vi "Initalize_33522b&2400&Delta_lxy.vi"(4 "Delta Mode Params In":T9={"High Level (A)"=0.001, "Low Level (A)"=-0.001, "Delay (s)"=0.002, "Num Cycles Mode"=enum."Finite Count", "Finite Count"=10, "Abort On\nCompliance?"=FALSE, "Cold Swithing\nMode Enabled?"=FALSE} {"Finite Count" min=1 max=65536; "Low Level (A)" min=-0.105 max=0.0 format="%.3p"; "High Level (A)" min=0.0 max=0.105 format="%.3p"; "Delay (s)" min=0.001 max=9999.999 format="%.3f"}, 5 "Output Level (0)":dbl=0.001, 6 "2812 -A Params In":T20={"Auto Range?"=FALSE, "Man / Selected\nRange"=enum."10mV", "Enable Digital\nFilter?"=FALSE, "Filter Type"=enum."Moving", "Filter Count"=10, "Filter\nWindow (%)"=0.01, "Enable Analog\nFilter?"=FALSE, "NPLCs"=5} {"Filter\nWindow (%)" min=0.0 max=10.0 step=0.01 format="%.2f"; "Filter Count" min=1 max=100; "NPLCs" min=1 max=10}, 7 "Compliance  Level (0.1)":dbl=10.0, 8 "error in (no error)":errorcluster, 11 "config":T1={"initialize"=enum."SR830", "6221"={"6221 Resource"="GPIB0::24::INSTR", "Delta status"=FALSE, "电流|RMS(A)"=0.0}, "SR830+6221"={"source"=0, "Current(A)"=0.0, "阻抗(Ohm)"=0.0, "SR830 1"=FALSE, "SR830 2"=FALSE, "SR830 3"=FALSE, "SR830 4"=FALSE, "VISA 1"="", "VISA 2"="", "VISA 3"="", "VISA 4"="", "Reserve 1"=0, "Reserve 2"=-1, "Reserve 3"=-1, "Reserve 4"=-1, "Sensitivity 1"=-1, "Sensitivity 2"=0, "Sensitivity 3"=-1, "Sensitivity 4"=-1, "量程入 1"=0, "量程入 2"=0, "量程入 3"=0, "量程入 4"=0}, "2400"={"2400"=FALSE, "VISA"="GPIB0::9::INSTR", "Output Level (0)"=1e-05, "Compliance  Level (0.1)"=10.0, "ch"=[]}, "ch"={"ch"=[], "current"=[], "change?"=[], "holding current\nwhen change ch?"=FALSE, "current offset"=[]}, "Instrument"={"limit"={"Field limit"=0.0, "Field rate limit"=0.0, "Temp limit"=0.0, "Temp low limit"=0.0, "Temp rate limit "=0.0}, "genarl"={"行数"=refnum, "编辑列表框？"=refnum, "列表框"=refnum, "camg 振荡状态"=refnum, "Aborting"=refnum, "数据文件"=refnum, "warning"=refnum, "vi路径"="", "Instrument Type"=enum."PPMS-Rotate"}, "cmag"={"TM620"="TCPIP0::192.168.1.5::4266::SOCKET", "M24C Resource"="GPIB0::24::INSTR", "4G supply"="", "Temp Status 24C"=refnum, "Temp"=refnum, "9T信号"=refnum, "4g supply status"=refnum, "in-plane"="", "out-plane"="", "in-plane signal"=FALSE, "out-plane signal"=FALSE, "in plane 信号"=refnum, "pzt volt"=refnum, "camg Rate"=refnum}, "lengtou2"={"750 visa"="", "750 rotate"="", "semaphore 340"=refnum, "semaphore 750"=refnum, "750 field status"=refnum, "Input (0:A) 340"=0, "340 Resource"="GPIB0::14::INSTR", "340 Status"=refnum, "Input (0:B) 340"=1, "Loop (0: 1)"=0, "Loop (1: 1)"=0, "TCP master instance"=refnum}, "lengtou"={"TCP master instance"=refnum, "335 Status"=refnum, "335 Resource "="GPIB0::24::INSTR", "Input (0:A) 335"=0, "Input (0:B) 335"=1, "Heater Output (1:1) 335"=1, "semaphore 335"=refnum}, "325 for test"={"quantum design"=refnum, "semaphore 325"=refnum, "325 Resource "="GPIB0::13::INSTR", "Input (0:A) 325"=0, "Heater Output (1:1) 325"=1, "325 Status"=refnum}}, "2614B"={"2614B chA"=FALSE, "2614B chB"=FALSE, "VISA"=""}, "33522b"={"33522b resource name"="GPIB0::16::INSTR", "零电压"=0.0, "最大电压"=148.0, "间隔"=4.0, "最小电压"=-48.0, "loop"=0.0}, "gating type"=enum."2614(daul)", "层数"=0, "行数"=0, "是否处理"=[], "current 2"=[]} {"Instrument"."325 for test"."Heater Output (1:1) 325" items=["1"=1, "2"=2]; "Instrument"."325 for test"."Input (0:A) 325" items=["A", "B"]; "Instrument"."lengtou"."Heater Output (1:1) 335" items=["1"=1, "2"=2]; "Instrument"."lengtou"."Input (0:B) 335" items=["A", "B"]; "Instrument"."lengtou"."Input (0:A) 335" items=["A", "B"]; "Instrument"."lengtou2"."Loop (1: 1)" items=["1", "2"]; "Instrument"."lengtou2"."Loop (0: 1)" items=["1", "2"]; "Instrument"."lengtou2"."Input (0:B) 340" items=["A", "B", "C", "D"]; "Instrument"."lengtou2"."Input (0:A) 340" items=["A", "B", "C", "D"]; "SR830+6221"."Sensitivity 4" items=["Auto Gain"=-1, "2 nV/fA"=0, "5 nV/fA"=1, "10 nV/fA"=2, "20 nV/fA"=3, "50 nV/fA"=4, "100 nV/fA"=5, "200 nV/fA"=6, "500 nV/fA"=7, "1 uV/pA"=8, "2 uV/pA"=9, "5 uV/pA"=10, "10 uV/pA"=11, "20 uV/pA"=12, "50 uV/pA"=13, "100 uV/pA"=14, "200 uV/pA"=15, "500 uV/pA"=16, "1 mV/nA"=17, "2 mV/nA"=18, "5 mV/nA"=19, "10 mV/nA"=20, "20 mV/nA"=21, "50 mV/nA"=22, "100 mV/nA"=23, "200 mV/nA"=24, "500 mV/mA"=25, "1 V/uA"=26]; "SR830+6221"."Sensitivity 3" items=["Auto Gain"=-1, "2 nV/fA"=0, "5 nV/fA"=1, "10 nV/fA"=2, "20 nV/fA"=3, "50 nV/fA"=4, "100 nV/fA"=5, "200 nV/fA"=6, "500 nV/fA"=7, "1 uV/pA"=8, "2 uV/pA"=9, "5 uV/pA"=10, "10 uV/pA"=11, "20 uV/pA"=12, "50 uV/pA"=13, "100 uV/pA"=14, "200 uV/pA"=15, "500 uV/pA"=16, "1 mV/nA"=17, "2 mV/nA"=18, "5 mV/nA"=19, "10 mV/nA"=20, "20 mV/nA"=21, "50 mV/nA"=22, "100 mV/nA"=23, "200 mV/nA"=24, "500 mV/mA"=25, "1 V/uA"=26]; "SR830+6221"."Sensitivity 1" items=["Auto Gain"=-1, "2 nV/fA"=0, "5 nV/fA"=1, "10 nV/fA"=2, "20 nV/fA"=3, "50 nV/fA"=4, "100 nV/fA"=5, "200 nV/fA"=6, "500 nV/fA"=7, "1 uV/pA"=8, "2 uV/pA"=9, "5 uV/pA"=10, "10 uV/pA"=11, "20 uV/pA"=12, "50 uV/pA"=13, "100 uV/pA"=14, "200 uV/pA"=15, "500 uV/pA"=16, "1 mV/nA"=17, "2 mV/nA"=18, "5 mV/nA"=19, "10 mV/nA"=20, "20 mV/nA"=21, "50 mV/nA"=22, "100 mV/nA"=23, "200 mV/nA"=24, "500 mV/mA"=25, "1 V/uA"=26]; "SR830+6221"."Sensitivity 2" items=["Auto Gain"=-1, "2 nV/fA"=0, "5 nV/fA"=1, "10 nV/fA"=2, "20 nV/fA"=3, "50 nV/fA"=4, "100 nV/fA"=5, "200 nV/fA"=6, "500 nV/fA"=7, "1 uV/pA"=8, "2 uV/pA"=9, "5 uV/pA"=10, "10 uV/pA"=11, "20 uV/pA"=12, "50 uV/pA"=13, "100 uV/pA"=14, "200 uV/pA"=15, "500 uV/pA"=16, "1 mV/nA"=17, "2 mV/nA"=18, "5 mV/nA"=19, "10 mV/nA"=20, "20 mV/nA"=21, "50 mV/nA"=22, "100 mV/nA"=23, "200 mV/nA"=24, "500 mV/mA"=25, "1 V/uA"=26]; "SR830+6221"."Reserve 4" items=["Auto Gain"=-1, "2 nV/fA"=0, "5 nV/fA"=1, "10 nV/fA"=2, "20 nV/fA"=3, "50 nV/fA"=4, "100 nV/fA"=5, "200 nV/fA"=6, "500 nV/fA"=7, "1 uV/pA"=8, "2 uV/pA"=9, "5 uV/pA"=10, "10 uV/pA"=11, "20 uV/pA"=12, "50 uV/pA"=13, "100 uV/pA"=14, "200 uV/pA"=15, "500 uV/pA"=16, "1 mV/nA"=17, "2 mV/nA"=18, "5 mV/nA"=19, "10 mV/nA"=20, "20 mV/nA"=21, "50 mV/nA"=22, "100 mV/nA"=23, "200 mV/nA"=24, "500 mV/mA"=25, "1 V/uA"=26]; "SR830+6221"."Reserve 3" items=["Auto Reserve"=-1, "High Reserve"=0, "Normal"=1, "Low Noise"=2]; "SR830+6221"."Reserve 2" items=["Auto Reserve"=-1, "High Reserve"=0, "Normal"=1, "Low Noise"=2]; "SR830+6221"."Reserve 1" items=["Auto Reserve"=-1, "High Reserve"=0, "Normal"=1, "Low Noise"=2]; "SR830+6221"."source" items=["SR830 1", "SR830 2", "SR830 3", "SR830 4"]}) -> (0 "输出簇":T1={"initialize"=enum."SR830", "6221"={"6221 Resource"="GPIB0::24::INSTR", "Delta status"=FALSE, "电流|RMS(A)"=0.0}, "SR830+6221"={"source"=0, "Current(A)"=0.0, "阻抗(Ohm)"=0.0, "SR830 1"=FALSE, "SR830 2"=FALSE, "SR830 3"=FALSE, "SR830 4"=FALSE, "VISA 1"="", "VISA 2"="", "VISA 3"="", "VISA 4"="", "Reserve 1"=0, "Reserve 2"=-1, "Reserve 3"=-1, "Reserve 4"=-1, "Sensitivity 1"=-1, "Sensitivity 2"=0, "Sensitivity 3"=-1, "Sensitivity 4"=-1, "量程入 1"=0, "量程入 2"=0, "量程入 3"=0, "量程入 4"=0}, "2400"={"2400"=FALSE, "VISA"="", "Output Level (0)"=1e-05, "Compliance  Level (0.1)"=10.0, "ch"=[]}, "ch"={"ch"=[], "current"=[], "change?"=[], "holding current\nwhen change ch?"=FALSE, "current offset"=[]}, "Instrument"={"limit"={"Field limit"=0.0, "Field rate limit"=0.0, "Temp limit"=0.0, "Temp low limit"=0.0, "Temp rate limit "=0.0}, "genarl"={"行数"=refnum, "编辑列表框？"=refnum, "列表框"=refnum, "camg 振荡状态"=refnum, "Aborting"=refnum, "数据文件"=refnum, "warning"=refnum, "vi路径"="", "Instrument Type"=enum."PPMS-Rotate"}, "cmag"={"TM620"="TCPIP0::192.168.1.5::4266::SOCKET", "M24C Resource"="GPIB0::24::INSTR", "4G supply"="", "Temp Status 24C"=refnum, "Temp"=refnum, "9T信号"=refnum, "4g supply status"=refnum, "in-plane"="", "out-plane"="", "in-plane signal"=FALSE, "out-plane signal"=FALSE, "in plane 信号"=refnum, "pzt volt"=refnum, "camg Rate"=refnum}, "lengtou2"={"750 visa"="", "750 rotate"="", "semaphore 340"=refnum, "semaphore 750"=refnum, "750 field status"=refnum, "Input (0:A) 340"=0, "340 Resource"="GPIB0::14::INSTR", "340 Status"=refnum, "Input (0:B) 340"=1, "Loop (0: 1)"=0, "Loop (1: 1)"=0, "TCP master instance"=refnum}, "lengtou"={"TCP master instance"=refnum, "335 Status"=refnum, "335 Resource "="GPIB0::24::INSTR", "Input (0:A) 335"=0, "Input (0:B) 335"=1, "Heater Output (1:1) 335"=1, "semaphore 335"=refnum}, "325 for test"={"quantum design"=refnum, "semaphore 325"=refnum, "325 Resource "="GPIB0::13::INSTR", "Input (0:A) 325"=0, "Heater Output (1:1) 325"=1, "325 Status"=refnum}}, "2614B"={"2614B chA"=FALSE, "2614B chB"=FALSE, "VISA"=""}, "33522b"={"33522b resource name"="", "零电压"=0.0, "最大电压"=148.0, "间隔"=4.0, "最小电压"=-48.0, "loop"=0.0}, "gating type"=enum."2614(daul)", "层数"=0, "行数"=0, "是否处理"=[], "current 2"=[]} {"Instrument"."325 for test"."Heater Output (1:1) 325" items=["1"=1, "2"=2]; "Instrument"."325 for test"."Input (0:A) 325" items=["A", "B"]; "Instrument"."lengtou"."Heater Output (1:1) 335" items=["1"=1, "2"=2]; "Instrument"."lengtou"."Input (0:B) 335" items=["A", "B"]; "Instrument"."lengtou"."Input (0:A) 335" items=["A", "B"]; "Instrument"."lengtou2"."Loop (1: 1)" items=["1", "2"]; "Instrument"."lengtou2"."Loop (0: 1)" items=["1", "2"]; "Instrument"."lengtou2"."Input (0:B) 340" items=["A", "B", "C", "D"]; "Instrument"."lengtou2"."Input (0:A) 340" items=["A", "B", "C", "D"]; "SR830+6221"."Sensitivity 4" items=["Auto Gain"=-1, "2 nV/fA"=0, "5 nV/fA"=1, "10 nV/fA"=2, "20 nV/fA"=3, "50 nV/fA"=4, "100 nV/fA"=5, "200 nV/fA"=6, "500 nV/fA"=7, "1 uV/pA"=8, "2 uV/pA"=9, "5 uV/pA"=10, "10 uV/pA"=11, "20 uV/pA"=12, "50 uV/pA"=13, "100 uV/pA"=14, "200 uV/pA"=15, "500 uV/pA"=16, "1 mV/nA"=17, "2 mV/nA"=18, "5 mV/nA"=19, "10 mV/nA"=20, "20 mV/nA"=21, "50 mV/nA"=22, "100 mV/nA"=23, "200 mV/nA"=24, "500 mV/mA"=25, "1 V/uA"=26]; "SR830+6221"."Sensitivity 3" items=["Auto Gain"=-1, "2 nV/fA"=0, "5 nV/fA"=1, "10 nV/fA"=2, "20 nV/fA"=3, "50 nV/fA"=4, "100 nV/fA"=5, "200 nV/fA"=6, "500 nV/fA"=7, "1 uV/pA"=8, "2 uV/pA"=9, "5 uV/pA"=10, "10 uV/pA"=11, "20 uV/pA"=12, "50 uV/pA"=13, "100 uV/pA"=14, "200 uV/pA"=15, "500 uV/pA"=16, "1 mV/nA"=17, "2 mV/nA"=18, "5 mV/nA"=19, "10 mV/nA"=20, "20 mV/nA"=21, "50 mV/nA"=22, "100 mV/nA"=23, "200 mV/nA"=24, "500 mV/mA"=25, "1 V/uA"=26]; "SR830+6221"."Sensitivity 1" items=["Auto Gain"=-1, "2 nV/fA"=0, "5 nV/fA"=1, "10 nV/fA"=2, "20 nV/fA"=3, "50 nV/fA"=4, "100 nV/fA"=5, "200 nV/fA"=6, "500 nV/fA"=7, "1 uV/pA"=8, "2 uV/pA"=9, "5 uV/pA"=10, "10 uV/pA"=11, "20 uV/pA"=12, "50 uV/pA"=13, "100 uV/pA"=14, "200 uV/pA"=15, "500 uV/pA"=16, "1 mV/nA"=17, "2 mV/nA"=18, "5 mV/nA"=19, "10 mV/nA"=20, "20 mV/nA"=21, "50 mV/nA"=22, "100 mV/nA"=23, "200 mV/nA"=24, "500 mV/mA"=25, "1 V/uA"=26]; "SR830+6221"."Sensitivity 2" items=["Auto Gain"=-1, "2 nV/fA"=0, "5 nV/fA"=1, "10 nV/fA"=2, "20 nV/fA"=3, "50 nV/fA"=4, "100 nV/fA"=5, "200 nV/fA"=6, "500 nV/fA"=7, "1 uV/pA"=8, "2 uV/pA"=9, "5 uV/pA"=10, "10 uV/pA"=11, "20 uV/pA"=12, "50 uV/pA"=13, "100 uV/pA"=14, "200 uV/pA"=15, "500 uV/pA"=16, "1 mV/nA"=17, "2 mV/nA"=18, "5 mV/nA"=19, "10 mV/nA"=20, "20 mV/nA"=21, "50 mV/nA"=22, "100 mV/nA"=23, "200 mV/nA"=24, "500 mV/mA"=25, "1 V/uA"=26]; "SR830+6221"."Reserve 4" items=["Auto Gain"=-1, "2 nV/fA"=0, "5 nV/fA"=1, "10 nV/fA"=2, "20 nV/fA"=3, "50 nV/fA"=4, "100 nV/fA"=5, "200 nV/fA"=6, "500 nV/fA"=7, "1 uV/pA"=8, "2 uV/pA"=9, "5 uV/pA"=10, "10 uV/pA"=11, "20 uV/pA"=12, "50 uV/pA"=13, "100 uV/pA"=14, "200 uV/pA"=15, "500 uV/pA"=16, "1 mV/nA"=17, "2 mV/nA"=18, "5 mV/nA"=19, "10 mV/nA"=20, "20 mV/nA"=21, "50 mV/nA"=22, "100 mV/nA"=23, "200 mV/nA"=24, "500 mV/mA"=25, "1 V/uA"=26]; "SR830+6221"."Reserve 3" items=["Auto Reserve"=-1, "High Reserve"=0, "Normal"=1, "Low Noise"=2]; "SR830+6221"."Reserve 2" items=["Auto Reserve"=-1, "High Reserve"=0, "Normal"=1, "Low Noise"=2]; "SR830+6221"."Reserve 1" items=["Auto Reserve"=-1, "High Reserve"=0, "Normal"=1, "Low Noise"=2]; "SR830+6221"."source" items=["SR830 1", "SR830 2", "SR830 3", "SR830 4"]}, 3 "33522b resource name":refnum<visa-resource-name>)   [LabVIEW 2019, in "nematic.lvlib"]
uses:
  nematic.lvlib
  lib/Keithley 622x/Configure/2182 -A/Low Level/Typedefs/KE2182 -- Voltage Ranges.ctl
  lib/Keithley 622x/Configure/2182 -A/Low Level/Typedefs/KE2182 -- Filter Type.ctl
  lib/Keithley 622x/Configure/2182 -A/Low Level/Typedefs/KE2182 -- Filter Count.ctl
  lib/Keithley 622x/Configure/2182 -A/Low Level/Typedefs/KE2182 -- Filter Window.ctl
  lib/Keithley 622x/Configure/2182 -A/Low Level/Typedefs/KE2182 -- NPLCs.ctl
  lib/Keithley 622x/Configure/Delta PDelta DCon Modes/Typedefs/KE622x -- Delta Mode Params.ctl
  lib/Keithley 622x/Configure/Delta PDelta DCon Modes/Low Level/Typedefs/KE622x -- Delta PDelta Mode High Level.ctl
  lib/Keithley 622x/Configure/Delta PDelta DCon Modes/Low Level/Typedefs/KE622x -- Delta PDelta Mode Low Level.ctl
  lib/Keithley 622x/Configure/Delta PDelta DCon Modes/Low Level/Typedefs/KE622x -- Delta DCon Mode Delay.ctl
  lib/Keithley 622x/Configure/Delta PDelta DCon Modes/Low Level/Typedefs/KE622x -- Delta PDelta Mode Num Cycles Mode.ctl
  lib/Keithley 622x/Configure/Delta PDelta DCon Modes/Low Level/Typedefs/KE622x -- Delta PDelta Mode Num Cycles.ctl
  ctl/config.ctl
  <vilib>/NI/Modbus Library/API/Master/Modbus Master.lvclass
  ctl/initialize.ctl
  ctl/Instrument.ctl
  ctl/limit.ctl
  ctl/warning.ctl
  ctl/Instrument Type.ctl
  ctl/335 state.ctl
  ctl/9T mag field stauts.ctl
  C:/Users/fuyang/Desktop/postdoctor/labview/labview-measure/lib/QDInstrument.dll
  lib/QDInstrument.dll
  ctl/Gating type.ctl
  lib/Keithley 622x/Configure/Units/Typedefs/KE622x -- Voltage Meas Units.ctl
  lib/Keithley 24XX/Keithley 24XX.lvlib
  lib/Keithley 622x/Keithley 622x.lvlib
panel:
  in  "Init Delta Meas? (T)":bool=TRUE
  in  "Enable Remote Sensing (T: Enable)":bool=TRUE
  in  "Serial Configuration":T8={"Baud Rate"=9600, "Parity"=0, "Data Bits"=8, "Stop Bits"=10, "Flow Control"=0} {"Flow Control" items=["None", "XON/XOFF", "RTS/CTS", "XON/XOFF & RTS/CTS", "DTR/DSR", "XON/XOFF & DTR/DSR"]; "Stop Bits" items=["1.0"=10, "1.5"=15, "2.0"=20]; "Data Bits" items=["7"=7, "8"=8]; "Parity" items=["None", "Odd", "Even", "Mark", "Space"]; "Baud Rate" items=["300"=300, "600"=600, "1200"=1200, "2400"=2400, "4800"=4800, "9600"=9600, "19200"=19200]}
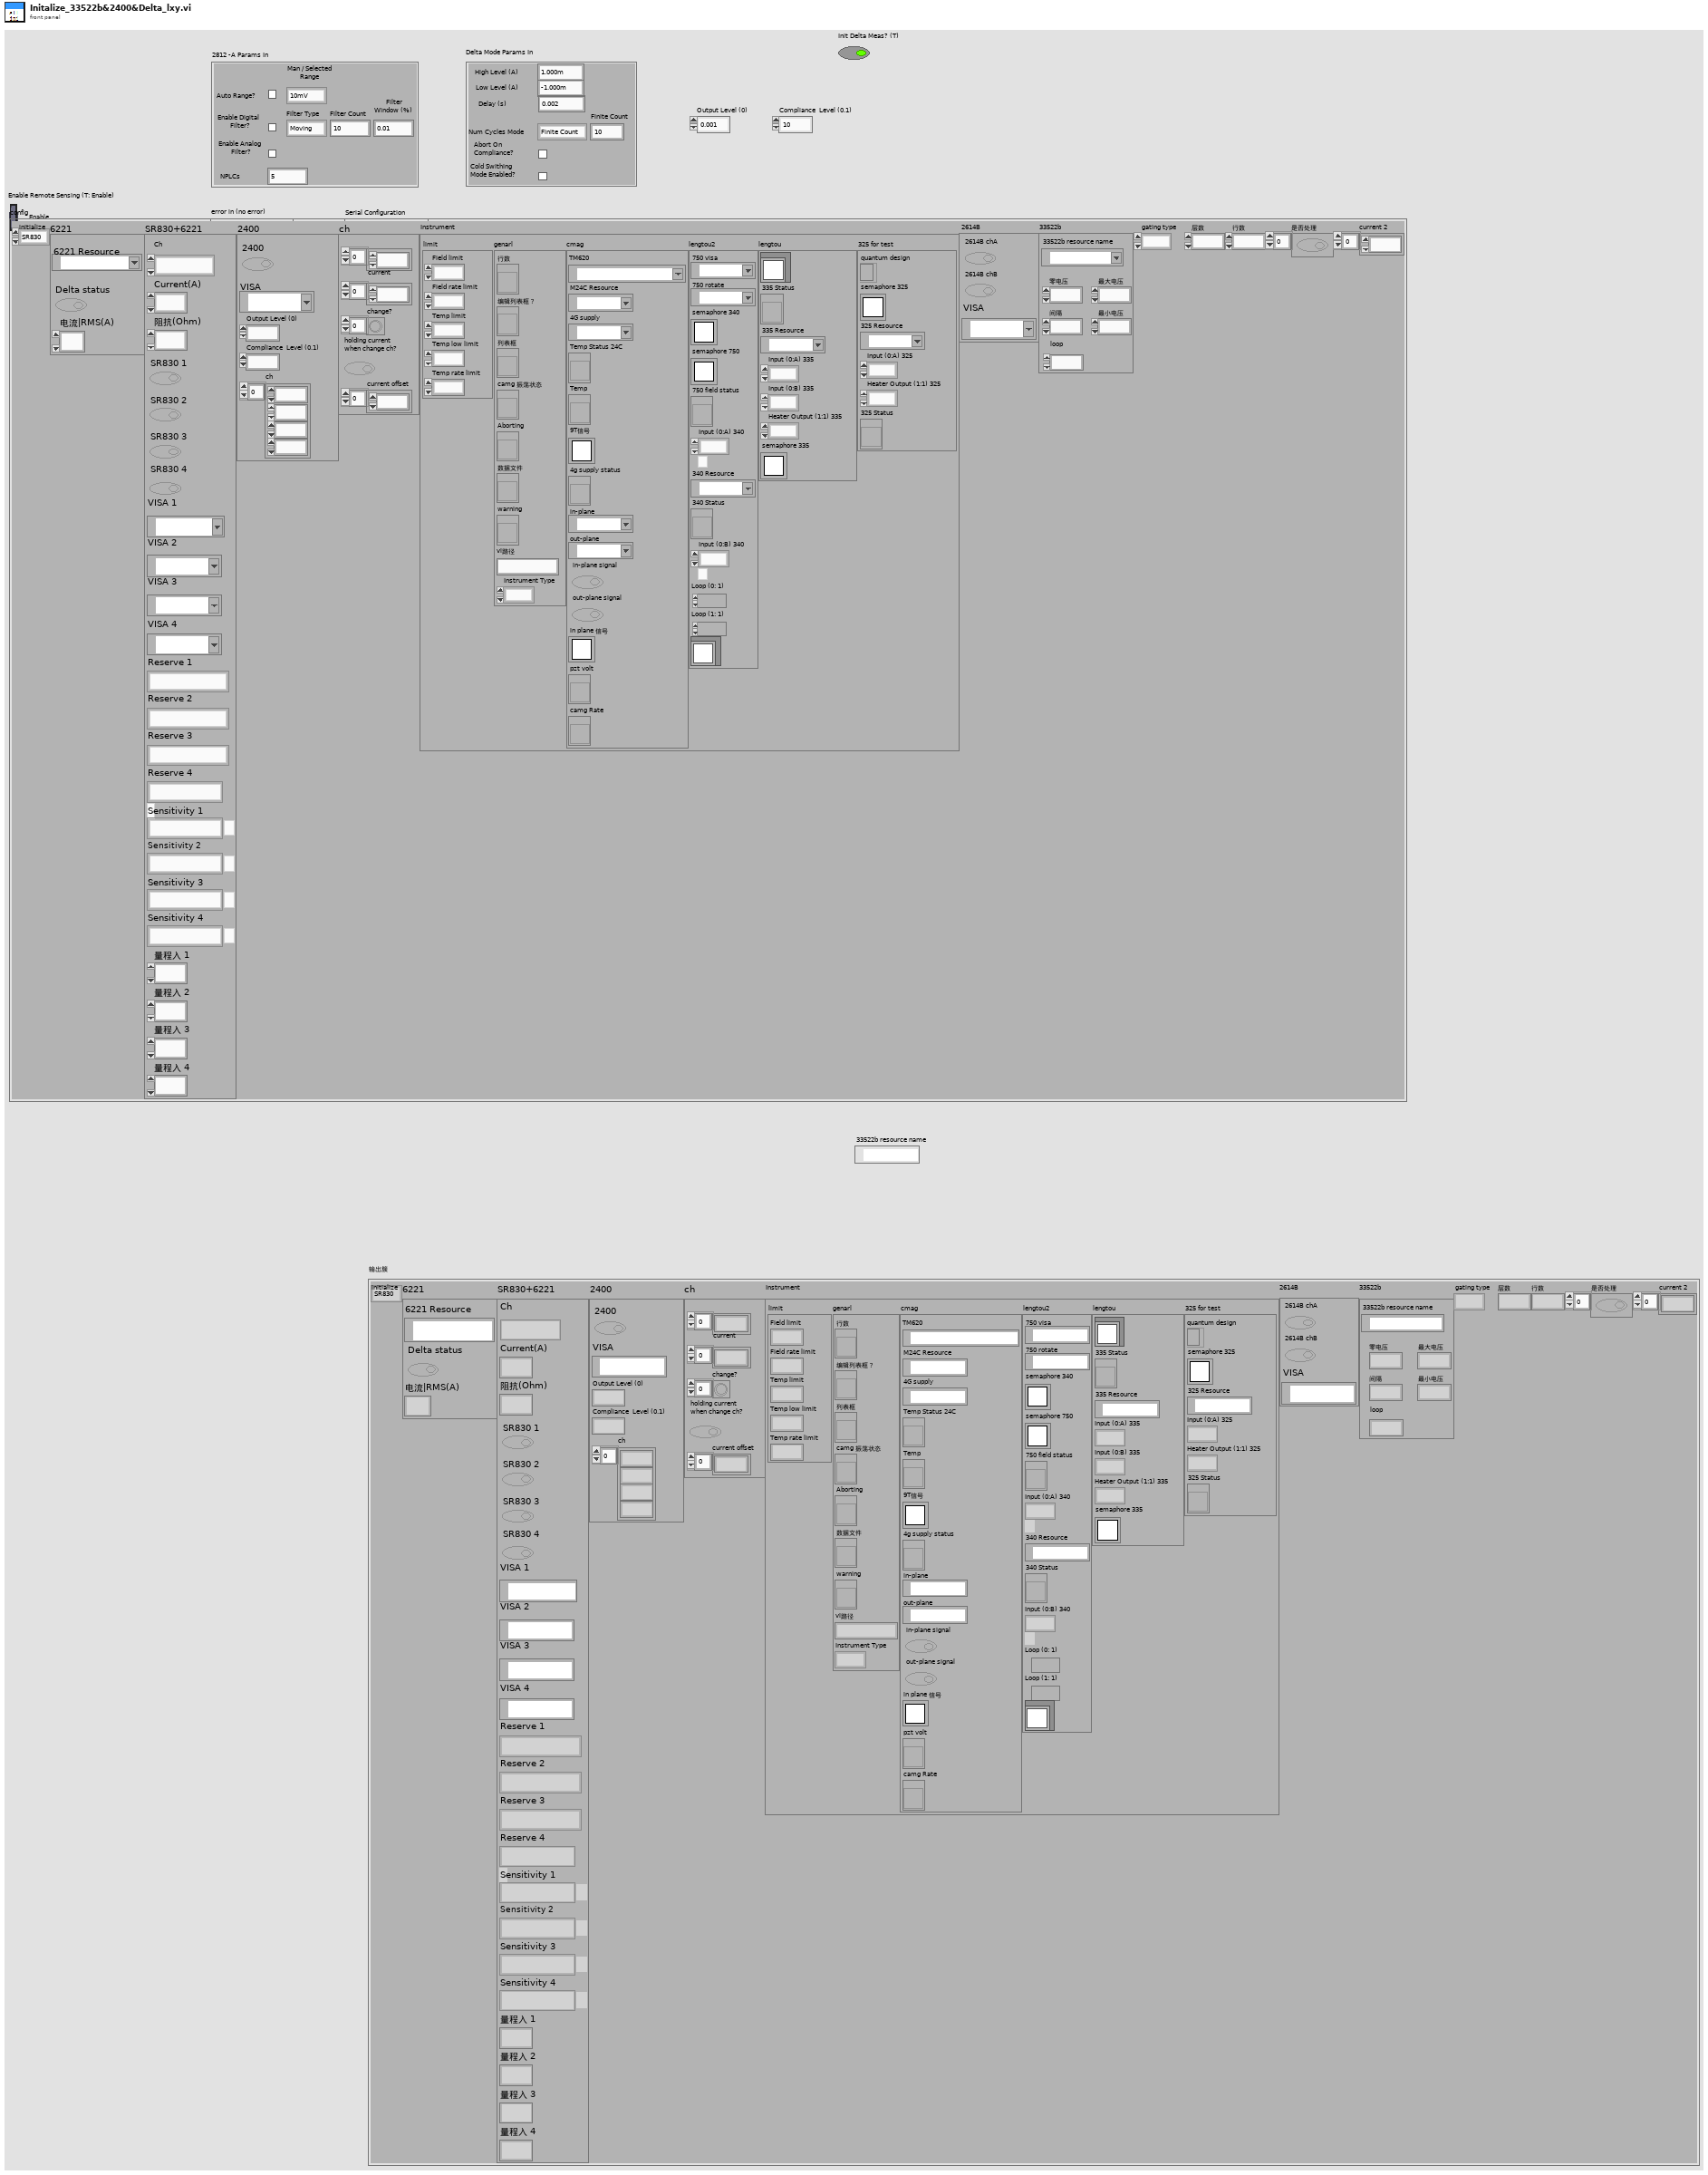
[diagram p1: front panel]
types:
  T1 = typedef "config.ctl" = cluster{"initialize":T2, "6221":cluster{"6221 Resource":refnum<visa-resource-name>, "Delta status":bool, "电流|RMS(A)":dbl}, "SR830+6221":cluster{"source":u16, "Current(A)":dbl, "阻抗(Ohm)":dbl, "SR830 1":bool, "SR830 2":bool, "SR830 3":bool, "SR830 4":bool, "VISA 1":refnum<visa-resource-name>, "VISA 2":refnum<visa-resource-name>, "VISA 3":refnum<visa-resource-name>, "VISA 4":refnum<visa-resource-name>, "Reserve 1":i16, "Reserve 2":i16, "Reserve 3":i16, "Reserve 4":i16, "Sensitivity 1":i16, "Sensitivity 2":i16, "Sensitivity 3":i16, "Sensitivity 4":i16, "量程入 1":i32, "量程入 2":i32, "量程入 3":i32, "量程入 4":i32}, "2400":cluster{"2400":bool, "VISA":refnum<visa-resource-name>, "Output Level (0)":dbl, "Compliance  Level (0.1)":dbl, "ch":i32[]}, "ch":cluster{"ch":i32[], "current":dbl[], "change?":bool[], "holding current\nwhen change ch?":bool, "current offset":dbl[]}, "Instrument":T3, "2614B":cluster{"2614B chA":bool, "2614B chB":bool, "VISA":refnum<visa-resource-name>}, "33522b":cluster{"33522b resource name":refnum<visa-resource-name>, "零电压":dbl, "最大电压":dbl, "间隔":dbl, "最小电压":dbl, "loop":dbl}, "gating type":T7, "层数":i32, "行数":i32, "是否处理":bool[], "current 2":dbl[]}
  T2 = typedef "initialize.ctl" = enum16{"SR830", "keithley6221-SR830", "Delta", "Delta-tunnelling", "keithley6221-2182-DC", "PZT", "4200"}
  T3 = typedef "Instrument.ctl" = cluster{"limit":T4, "genarl":cluster{"行数":refnum<vi>, "编辑列表框？":refnum<vi>, "列表框":refnum<vi>, "camg 振荡状态":refnum<vi>, "Aborting":refnum<vi>, "数据文件":refnum<vi>, "warning":refnum<vi>, "vi路径":string, "Instrument Type":T5}, "cmag":cluster{"TM620":refnum<visa-resource-name>, "M24C Resource":refnum<visa-resource-name>, "4G supply":refnum<visa-resource-name>, "Temp Status 24C":refnum<vi>, "Temp":refnum<vi>, "9T信号":T6, "4g supply status":refnum<vi>, "in-plane":refnum<visa-resource-name>, "out-plane":refnum<visa-resource-name>, "in-plane signal":bool, "out-plane signal":bool, "in plane 信号":T6, "pzt volt":refnum<vi>, "camg Rate":refnum<vi>}, "lengtou2":cluster{"750 visa":refnum<visa-resource-name>, "750 rotate":refnum<visa-resource-name>, "semaphore 340":T6, "semaphore 750":T6, "750 field status":refnum<vi>, "Input (0:A) 340":u16, "340 Resource":refnum<visa-resource-name>, "340 Status":refnum<vi>, "Input (0:B) 340":u16, "Loop (0: 1)":u16, "Loop (1: 1)":u16, "TCP master instance":refnum<class "Modbus Master.lvclass">}, "lengtou":cluster{"TCP master instance":refnum<class "Modbus Master.lvclass">, "335 Status":refnum<vi>, "335 Resource ":refnum<visa-resource-name>, "Input (0:A) 335":u16, "Input (0:B) 335":u16, "Heater Output (1:1) 335":u16, "semaphore 335":T6}, "325 for test":cluster{"quantum design":refnum<k24>, "semaphore 325":T6, "325 Resource ":refnum<visa-resource-name>, "Input (0:A) 325":u16, "Heater Output (1:1) 325":u16, "325 Status":refnum<vi>}}
  T4 = typedef "limit.ctl" = cluster{"Field limit":dbl, "Field rate limit":dbl, "Temp limit":dbl, "Temp low limit":dbl, "Temp rate limit ":dbl}
  T5 = typedef "Instrument Type.ctl" = enum16{"PPMS", "VersaLab", "DynaCool", "SVSM", "PPMS-Rotate", "Lakeshore335", "lengtou2", "9T mag old", "9T cmag", "9T cmag DAC", "9T cmag rotate", "test"}
  T6 = typedef "Semaphore RefNum" = refnum<k1>
  T7 = typedef "Gating type.ctl" = enum32{"null", "2614(daul)", "2400", "6517B"}
  T8 = cluster{"Baud Rate":u32, "Parity":u16, "Data Bits":u16, "Stop Bits":u16, "Flow Control":u16}
  T9 = typedef "Keithley 622x.lvlib/KE622x -- Delta Mode Params.ctl" = cluster{"High Level (A)":T10, "Low Level (A)":T11, "Delay (s)":T12, "Num Cycles Mode":T13, "Finite Count":T14, "Abort On\nCompliance?":bool, "Cold Swithing\nMode Enabled?":bool}
  T10 = typedef "Keithley 622x.lvlib/KE622x -- Delta PDelta Mode High Level.ctl" = dbl
  T11 = typedef "Keithley 622x.lvlib/KE622x -- Delta PDelta Mode Low Level.ctl" = dbl
  T12 = typedef "Keithley 622x.lvlib/KE622x -- Delta DCon Mode Delay.ctl" = dbl
  T13 = typedef "Keithley 622x.lvlib/KE622x -- Delta PDelta Mode Num Cycles Mode.ctl" = enum16{"Finite Count", "Infinite"}
  T14 = typedef "Keithley 622x.lvlib/KE622x -- Delta PDelta Mode Num Cycles.ctl" = u32
  T15 = typedef "Keithley 622x.lvlib/KE2182 -- Voltage Ranges.ctl" = enum16{"10mV", "100mV", "1V", "10V", "100V"}
  T16 = typedef "Keithley 622x.lvlib/KE2182 -- Filter Type.ctl" = enum16{"Moving", "Repeat"}
  T17 = typedef "Keithley 622x.lvlib/KE2182 -- Filter Count.ctl" = u32
  T18 = typedef "Keithley 622x.lvlib/KE2182 -- Filter Window.ctl" = dbl
  T19 = typedef "Keithley 622x.lvlib/KE2182 -- NPLCs.ctl" = u32
  T20 = cluster{"Auto Range?":bool, "Man / Selected\nRange":T15, "Enable Digital\nFilter?":bool, "Filter Type":T16, "Filter Count":T17, "Filter\nWindow (%)":T18, "Enable Analog\nFilter?":bool, "NPLCs":T19}
  T21 = typedef "Keithley 622x.lvlib/KE622x -- Voltage Meas Units.ctl" = enum16{"Volts", "Ohms", "Watts", "Siemens"}
  T22 = typedef "Keithley 622x.lvlib/KE622x -- On Off Control.ctl" = enum16{"Off", "On"}
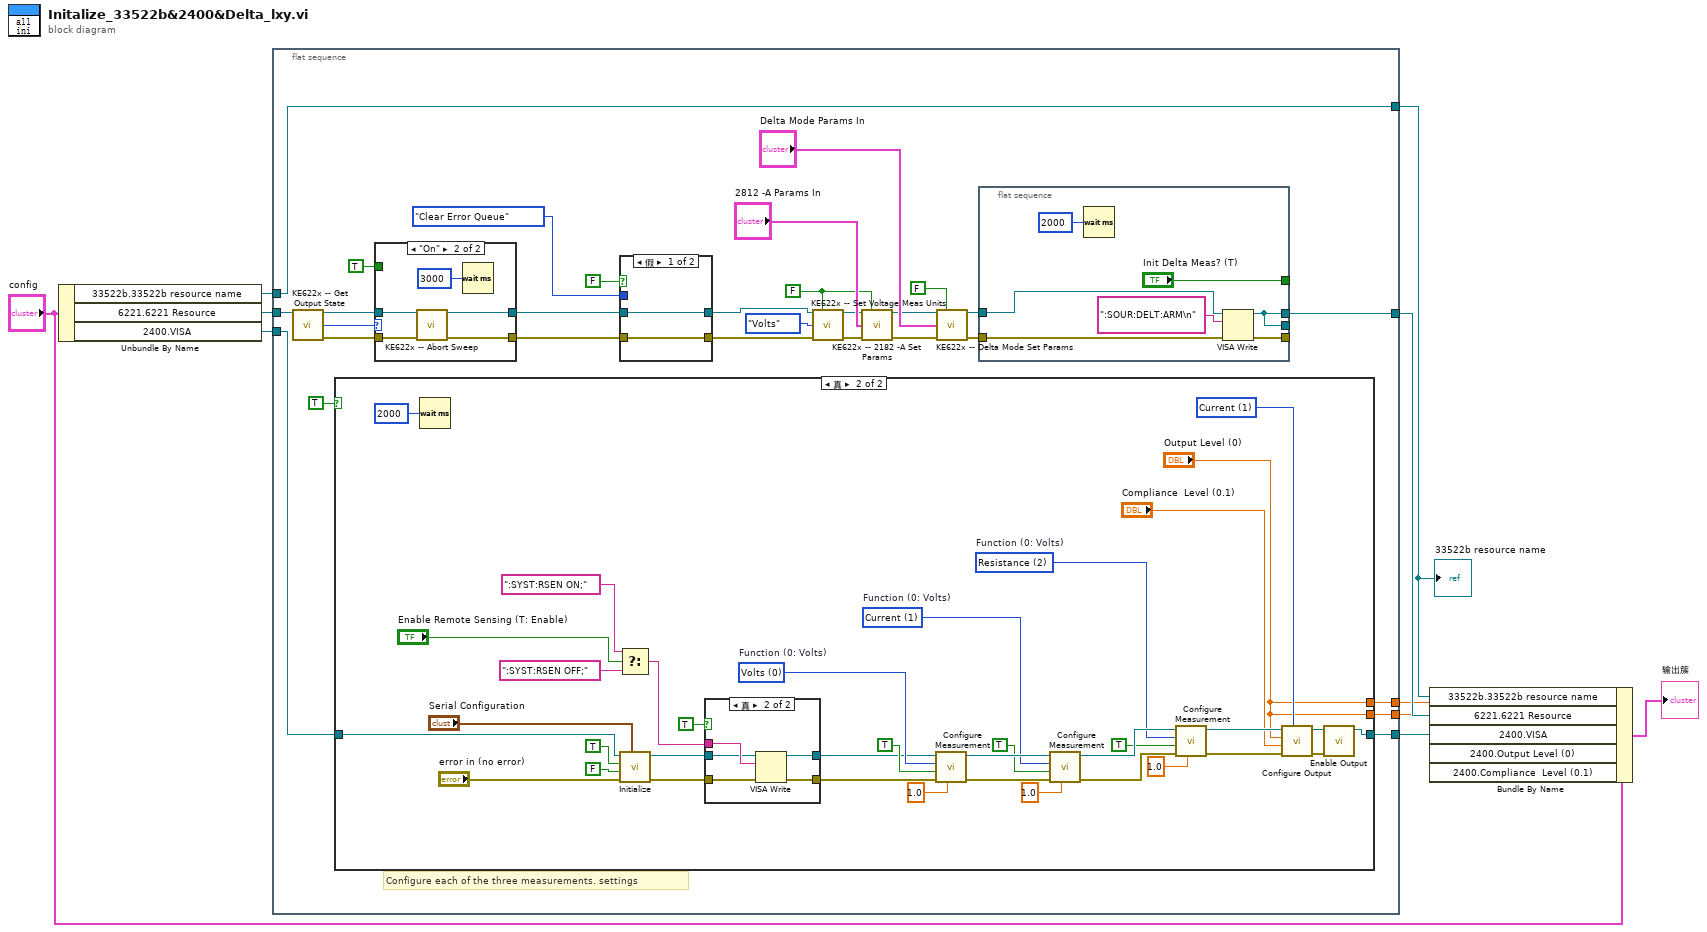
[diagram p0: block diagram]
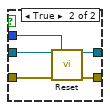
[diagram p4: hidden frame]
diagram:
  n1 = Unbundle By Name("config") -> ("33522b.33522b resource name"=w10:refnum<visa-resource-name>, "6221.6221 Resource"=w9:refnum<visa-resource-name>, "2400.VISA"=w8:refnum<visa-resource-name>)
  n2 = flat-sequence {
    tunnel: [w39] -> w7
    tunnel: [w38] -> w6
    tunnel: [w37] -> w5
    tunnel: w8 -> [w16]
    tunnel: w9 -> [w18]
    tunnel: w10 -> [w39]
    tunnel: [w12] -> w2
    tunnel: [w11] -> w1
    frame #0 {
      w15 = FALSE ("Check For SCPI Errors? (T)")
      # "Configure each of the three measurements. settings"
      n3 = call "KE622x -- Get Output State.vi"("Resource In"=w18) -> ("Resource Out (dupl)"=w24:refnum<visa-resource-name>, "Output State"=w26:T22, "error out"=w25:errorcluster)  [unwired: 12 in]
      n4 = case shown="真" TRUE {
        tunnel: w16 -> [w47 w71]
        tunnel: [w47 w54] -> w37
        tunnel: [_ "Output Level (0)"] -> w12
        tunnel: [_ "Output Level (0)"] -> w11
        frame False {
        }
        frame True {
          w57 = u16 1 items=["Voltage", "Current"] ("Source Mode  (0: Voltage)")
          w77 = u16 2 items=["Volts", "Current", "Resistance"]  # Function (0: Volts)
          w78 = u16 1 items=["Volts", "Current", "Resistance"]  # Function (0: Volts)
          w79 = u16 0 items=["Volts", "Current", "Resistance"]  # Function (0: Volts)
          n5 = Wait (ms)(milliseconds to wait=u32 2000) -> ()  [unwired: 1 out]
          n6 = Select(t=":SYST:RSEN ON;", s="Enable Remote Sensing (T: Enable)", f=":SYST:RSEN OFF;") -> (s? t:f=w61:string)
          n7 = call "Initialize.vi"("Serial Configuration"="Serial Configuration", "error in (no error)"="error in (no error)", "Reset (True)"=FALSE, "ID Query (True)"=TRUE, "VISA resource name"=w71) -> ("error out"=w49:errorcluster, "VISA resource name out"=w50:refnum<visa-resource-name>)  [unwired: 5 in]
          n8 = case shown="真" TRUE {
            tunnel: w61 -> [_ w90]
            tunnel: [w85 w89] -> w52
            tunnel: [w84 w88] -> w51
            tunnel: w50 -> [w85 w87]
            tunnel: w49 -> [w84 w86]
            frame False {
            }
            frame True {
              n9 = VISA Write(VISA resource name=w87, write buffer=w90, error in (no error)=w86) -> (VISA resource name out=w89:refnum<visa-resource-name>, error out=w88:errorcluster)  [unwired: 1 out]
            }
          }
          n10 = call "Configure Measurement.vi"("Manual Range (1.0)"=1.0 ("Voltage Manual Range (1.0)"), "error in (no error)"=w51, "Enable Auto Range (T:Enable)"=TRUE ("Enable Voltage Auto Range (T:Enable)"), "Function (0: Volts)"=w79, "VISA resource name"=w52) -> ("error out"=w82:errorcluster, "VISA resource name out"=w83:refnum<visa-resource-name>)  [unwired: 5 in]
          n11 = call "Configure Measurement.vi"("Manual Range (1.0)"=1.0 ("Current Manual Range (1.0)"), "error in (no error)"=w82, "Enable Auto Range (T:Enable)"=TRUE ("Enable Current Auto Range (T:Enable)"), "Function (0: Volts)"=w78, "VISA resource name"=w83) -> ("error out"=w81:errorcluster, "VISA resource name out"=w80:refnum<visa-resource-name>)  [unwired: 5 in]
          n12 = call "Configure Measurement.vi"("Manual Range (1.0)"=1.0 ("Resistance Manual Range (1.0)"), "error in (no error)"=w81, "Enable Auto Range (T:Enable)"=TRUE ("Enable Resistance Auto Range (T:Enable)"), "Function (0: Volts)"=w77, "VISA resource name"=w80) -> ("error out"=w59:errorcluster, "VISA resource name out"=w60:refnum<visa-resource-name>)  [unwired: 5 in]
          n13 = call "Configure Output.vi"("Source Mode  (0: Voltage)"=w57, "error in (no error)"=w59, "Compliance  Level (0.1)"="Compliance  Level (0.1)", "Output Level (0)"="Output Level (0)", "VISA resource name"=w60) -> ("error out"=w55:errorcluster, "VISA resource name out"=w56:refnum<visa-resource-name>)  [unwired: 5 in]
          n14 = call "Enable Output.vi"("error in (no error)"=w55, "VISA resource name"=w56) -> ("VISA resource name out"=w54:refnum<visa-resource-name>)  [unwired: 8 in, 1 out]
        }
      }
      n15 = case shown="\"On\"" w26 {
        tunnel: w24 -> [w99 w103]
        tunnel: [w99 w102] -> w33
        tunnel: w25 -> [w98 w101]
        tunnel: [w98 w100] -> w34
        tunnel: TRUE -> [_ _]
        frame "Off", Default {
        }
        frame "On" {
          n16 = call "KE622x -- Abort Sweep.vi"("Resource In"=w103, "error in (no error)"=w101) -> ("Resource Out (dupl)"=w102:refnum<visa-resource-name>, "error out"=w100:errorcluster)  [unwired: 12 in]
          n17 = Wait (ms)(milliseconds to wait=u32 3000 ("等待时间（毫秒）")) -> ()  [unwired: 1 out]
        }
      }
      n18 = case shown="假" FALSE {
        tunnel: w33 -> [w92 w97]
        tunnel: enum16{"Clear Error Queue", "Error Query"}."Clear Error Queue" ("Error Queue Option") -> [_ w96]
        tunnel: [w92 w95] -> w28
        tunnel: w34 -> [w91 w94]
        tunnel: [w91 w93] -> w30
        frame False {
        }
        frame True {
          n19 = call "Reset.vi"("VISA resource name"=w97, "Error Queue Option"=w96, "error in (no error)"=w94) -> ("VISA resource name out"=w95:refnum<visa-resource-name>, "error out"=w93:errorcluster)  [unwired: 11 in]
        }
      }
      n20 = call "KE622x -- Set Voltage Meas Units.vi"("Resource In"=w28, "Check For SCPI Errors? (T)"=w15, "Voltage Meas Units"=KE622x_--_Voltage_Meas_Units."Volts", "error in (no error)"=w30) -> ("Resource Out (dupl)"=w27:refnum<visa-resource-name>, "error out"=w31:errorcluster)  [unwired: 10 in]
      n21 = call "KE622x -- 2182 -A Set Params.vi"("622x Resource In"=w27, "Check For SCPI Errors? (T)"=w15, "2812 -A Params In"="2812 -A Params In", "error in (no error)"=w31) -> ("622x Resource Out (dupl)"=w29:refnum<visa-resource-name>, "error out"=w32:errorcluster)  [unwired: 9 in, 1 out]
      n22 = call "KE622x -- Delta Mode Set Params.vi"("Resource In"=w29, "Check For SCPI Errors? (T)"=FALSE, "Delta Mode Params In"="Delta Mode Params In", "error in (no error)"=w32) -> ("Resource Out (dupl)"=w14:refnum<visa-resource-name>, "error out"=w13:errorcluster)  [unwired: 9 in, 1 out]
      n23 = flat-sequence {
        tunnel: w13 -> [w45]
        tunnel: w14 -> [w44]
        tunnel: ["Init Delta Meas? (T)"] -> _
        tunnel: [w40] -> _
        tunnel: [w42] -> _
        tunnel: [w40] -> w38
        frame #0 {
          n24 = Wait (ms)(milliseconds to wait=u32 2000) -> ()  [unwired: 1 out]
          n25 = VISA Write(VISA resource name=w44, write buffer=":SOUR:DELT:ARM\n" ("format string"), error in (no error)=w45) -> (VISA resource name out=w40:refnum<visa-resource-name>, error out=w42:errorcluster)  [unwired: 1 out]
        }
      }
    }
  }
  n26 = Bundle By Name(cluster="config", "33522b.33522b resource name"=w7, "6221.6221 Resource"=w6, "2400.VISA"=w5, "2400.Output Level (0)"=w2, "2400.Compliance  Level (0.1)"=w1) -> (→"输出簇":T1)
  "33522b resource name" <- w7
